vi "9. SCADA_Robotic_Arm_5.vi"() -> ()   [LabVIEW 2020]
panel:
  out "Truck Move":dbl(slide) scale=0.0..100.0
  out "Counter":dbl
  out "Conveyor_Belt":dbl(slide) scale=0.0..10.0
  out "Bottle in Truck":bool
  in  "Numeric":dbl
  in  "stop":bool
  in  "?":enum32{"Control Panel"}(tab)
  in  "LEFT/RIGHT":dbl(slide) scale=0.0..500.0
  in  "UP/DOWN":dbl(slide) scale=157.0..420.0
  in  "Conveyor_ON/OFF":bool
  in  "CONVEYOR_\nCONTROL":dbl(slide) scale=0.0..10.0
  in  "New Bottle":bool
  in  "Bottle Pic":bool
  in  "Bottle In Truck":i32(slide) scale=430.0..554.0
  in  "Truck Move":dbl(slide) scale=0.0..100.0
  out "Boolean":bool
  out "Bottle":bool
  # "Counter"
  # "Conveyor_Belt"
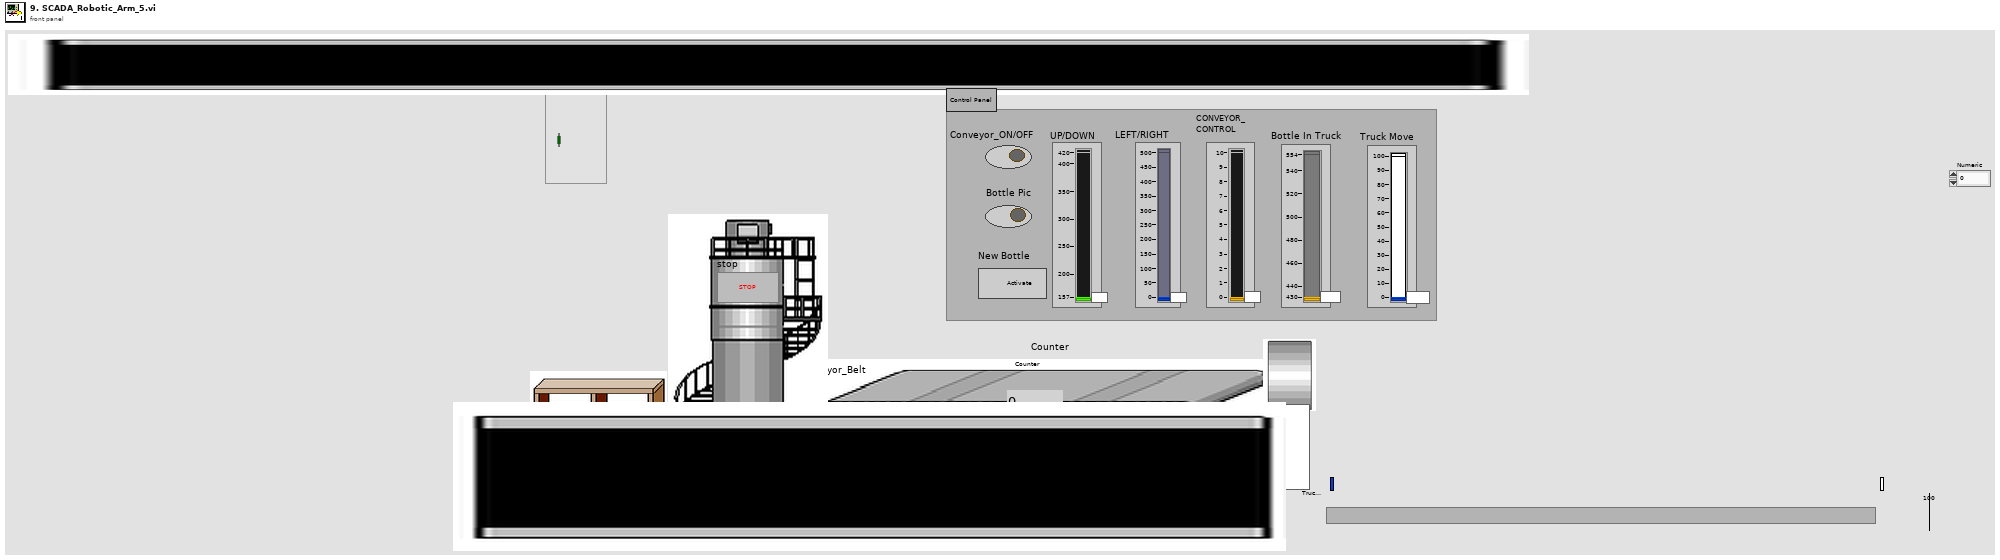
[diagram p1: front panel]
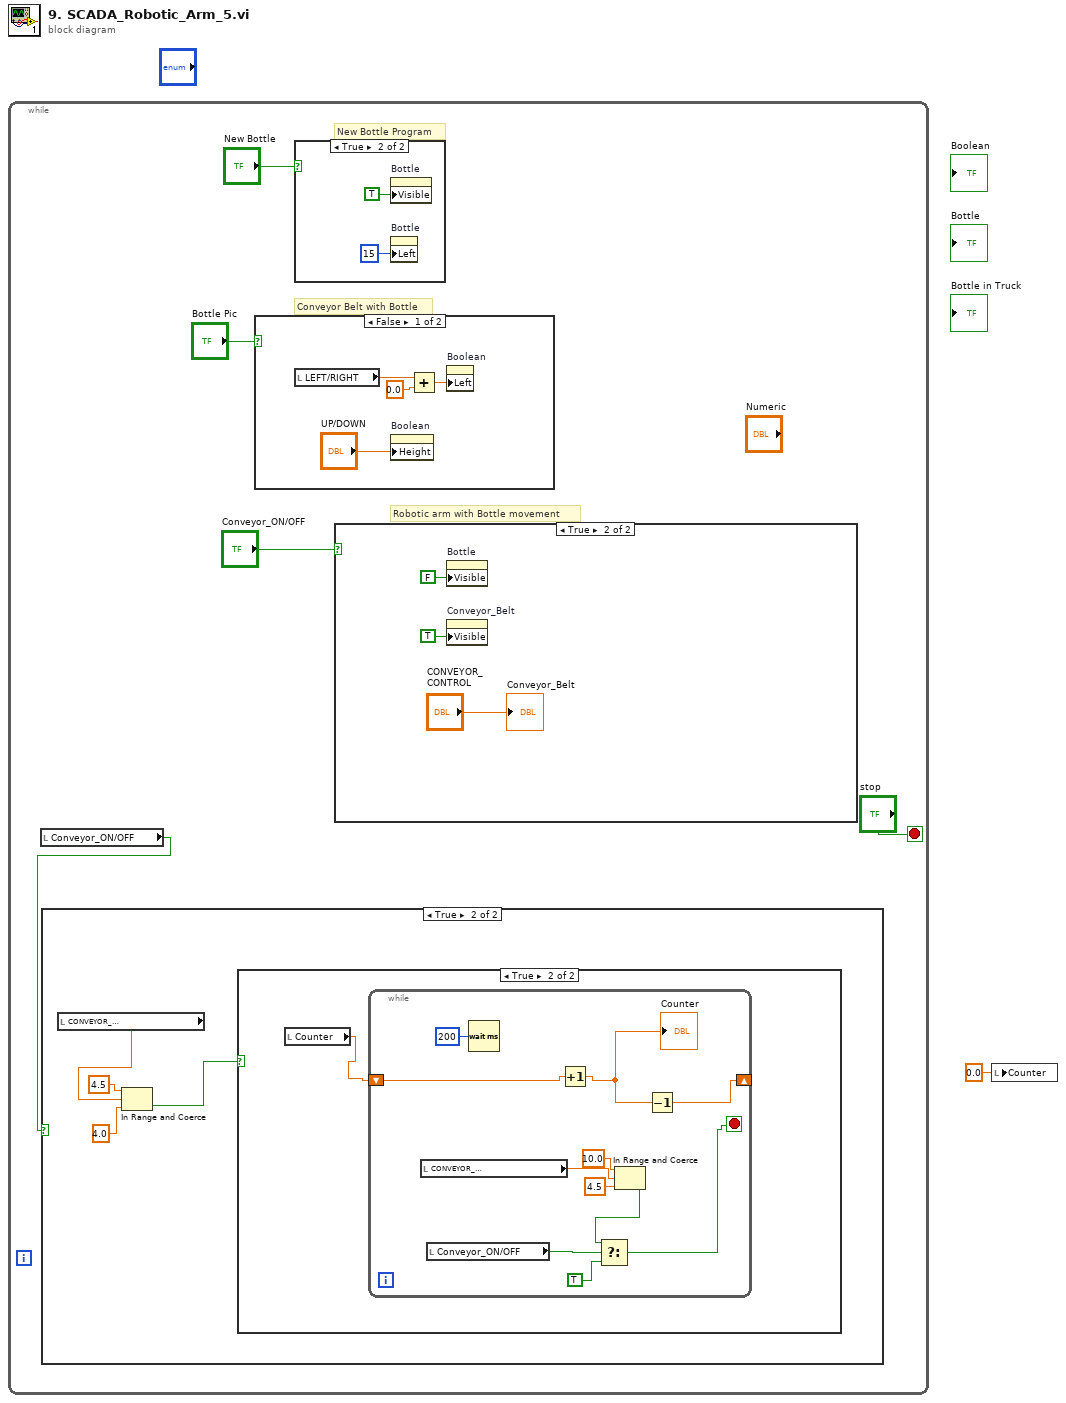
[diagram p0: block diagram]
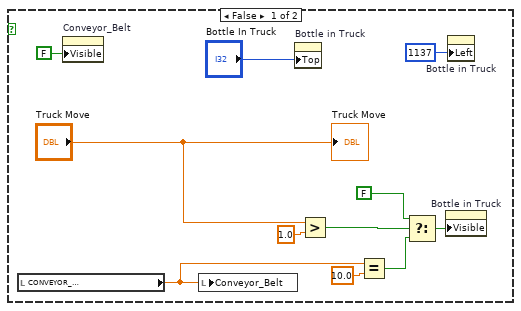
[diagram p5: hidden frame]
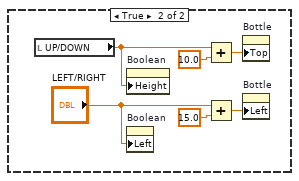
[diagram p6: hidden frame]
diagram:
  n1 = while {
    stop <- "stop" stop-if-true
    # "Conveyor Belt with Bottle"
    # "Robotic arm with Bottle movement"
    # "New Bottle Program"
    n2 = local read "Conveyor_ON/OFF"() -> (w2:bool)
    n3 = case shown="True" w2 {
      frame False {
      }
      frame True {
        n4 = local read "CONVEYOR_\nCONTROL"() -> (w10:dbl)
        n5 = In Range and Coerce(upper limit=4.5, x=w10, lower limit=4.0) -> (In Range?=w7:bool)  [unwired: 1 out]
        n6 = case shown="True" w7 {
          frame False {
          }
          frame True {
            n7 = local read "Counter"() -> (w11:dbl)
            n8 = while {
              shift-right: [w13] -> _
              shift-left: w11 -> [w22]
              stop <- w16 stop-if-true
              n9 = local read "CONVEYOR_\nCONTROL"() -> (w21:dbl)
              n10 = local read "Conveyor_ON/OFF"() -> (w18:bool)
              n11 = Wait (ms)(milliseconds to wait=u32 200) -> ()  [unwired: 1 out]
              n12 = Increment(x=w22) -> (x+1=w12:dbl)
              "Counter" <- w12
              n13 = In Range and Coerce(upper limit=10.0, x=w21, lower limit=4.5) -> (In Range?=w17:bool)  [unwired: 1 out]
              n14 = Select(t=w17, s=w18, f=TRUE) -> (s? t:f=w16:bool)
              n15 = Decrement(x=w12) -> (x-1=w13:dbl)
            }
          }
        }
      }
    }
    n16 = case shown="False" "Bottle Pic" {
      frame False {
        n17 = local read "LEFT/RIGHT"() -> (w40:dbl)
        n18 = property on="Boolean" class="Bool (strict)"("Height"="UP/DOWN") -> ()  [unwired: 2 in, 2 out]
        n19 = Add(x=w40, y=0.0) -> (x+y=w39:dbl)
        n20 = property on="Boolean" class="Bool (strict)"("Left"=w39) -> ()  [unwired: 2 in, 2 out]
      }
      frame True {
        n21 = local read "UP/DOWN"() -> (w48:dbl)
        n22 = property on="Boolean" class="Bool (strict)"("Height"=w48) -> ()  [unwired: 2 in, 2 out]
        n23 = property on="Boolean" class="Bool (strict)"("Left"="LEFT/RIGHT") -> ()  [unwired: 2 in, 2 out]
        n24 = Add(x=w48, y=10.0) -> (x+y=w47:dbl)
        n25 = Add(x="LEFT/RIGHT", y=15.0) -> (x+y=w45:dbl)
        n26 = property on="Bottle" class="Bool (strict)"("Top"=w47) -> ()  [unwired: 2 in, 2 out]
        n27 = property on="Bottle" class="Bool (strict)"("Left"=w45) -> ()  [unwired: 2 in, 2 out]
      }
    }
    n28 = case shown="True" "New Bottle" {
      frame False {
      }
      frame True {
        n29 = property on="Bottle" class="Bool (strict)"("Visible"=TRUE) -> ()  [unwired: 2 in, 2 out]
        n30 = property on="Bottle" class="Bool (strict)"("Left"=15 ("Position:Left")) -> ()  [unwired: 2 in, 2 out]
      }
    }
    n31 = case shown="True" "Conveyor_ON/OFF" {
      frame False {
        n32 = local read "CONVEYOR_\nCONTROL"() -> (w33:dbl)
        n33 = property on="Conveyor_Belt" class="Slide (strict)"("Visible"=FALSE) -> ()  [unwired: 2 in, 2 out]
        n34 = local write "Conveyor_Belt"(w33) -> ()
        n35 = property on="Bottle in Truck" class="Bool (strict)"("Top"="Bottle In Truck") -> ()  [unwired: 2 in, 2 out]
        n36 = Greater?(x="Truck Move", y=1.0) -> (0:w28:bool)
        n37 = Equal?(x=w33, y=10.0) -> (x = y?=w26:bool)
        n38 = Select(t=FALSE, s=w28, f=w26) -> (s? t:f=w27:bool)
        n39 = property on="Bottle in Truck" class="Bool (strict)"("Visible"=w27) -> ()  [unwired: 2 in, 2 out]
        n40 = property on="Bottle in Truck" class="Bool (strict)"("Left"=1137 ("Position:Top")) -> ()  [unwired: 2 in, 2 out]
        "Truck Move" <- "Truck Move"
      }
      frame True {
        n41 = property on="Bottle" class="Bool (strict)"("Visible"=FALSE) -> ()  [unwired: 2 in, 2 out]
        n42 = property on="Conveyor_Belt" class="Slide (strict)"("Visible"=TRUE) -> ()  [unwired: 2 in, 2 out]
        "Conveyor_Belt" <- "CONVEYOR_\nCONTROL"
      }
    }
  }
  n43 = local write "Counter"(0.0 ("Counter")) -> ()
